vi "choose worker.vi"(9 "total":i32, 10 "Python version":string, 11 "user.xls path":path) -> ()   [LabVIEW 2020]
uses:
  status/emergency stop.vi
  status/experiment_No.vi
  status/status of worker1.vi
  status/pause1.vi
  status/status of worker2.vi
  status/pause2.vi
  status/status of worker3.vi
  status/pause3.vi
  status/pause4.vi
  status/status of worker4.vi
  status/stop software.vi
panel:
  in  "?":bool
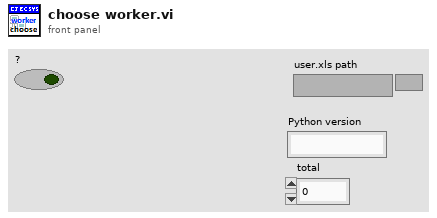
[diagram p1: front panel]
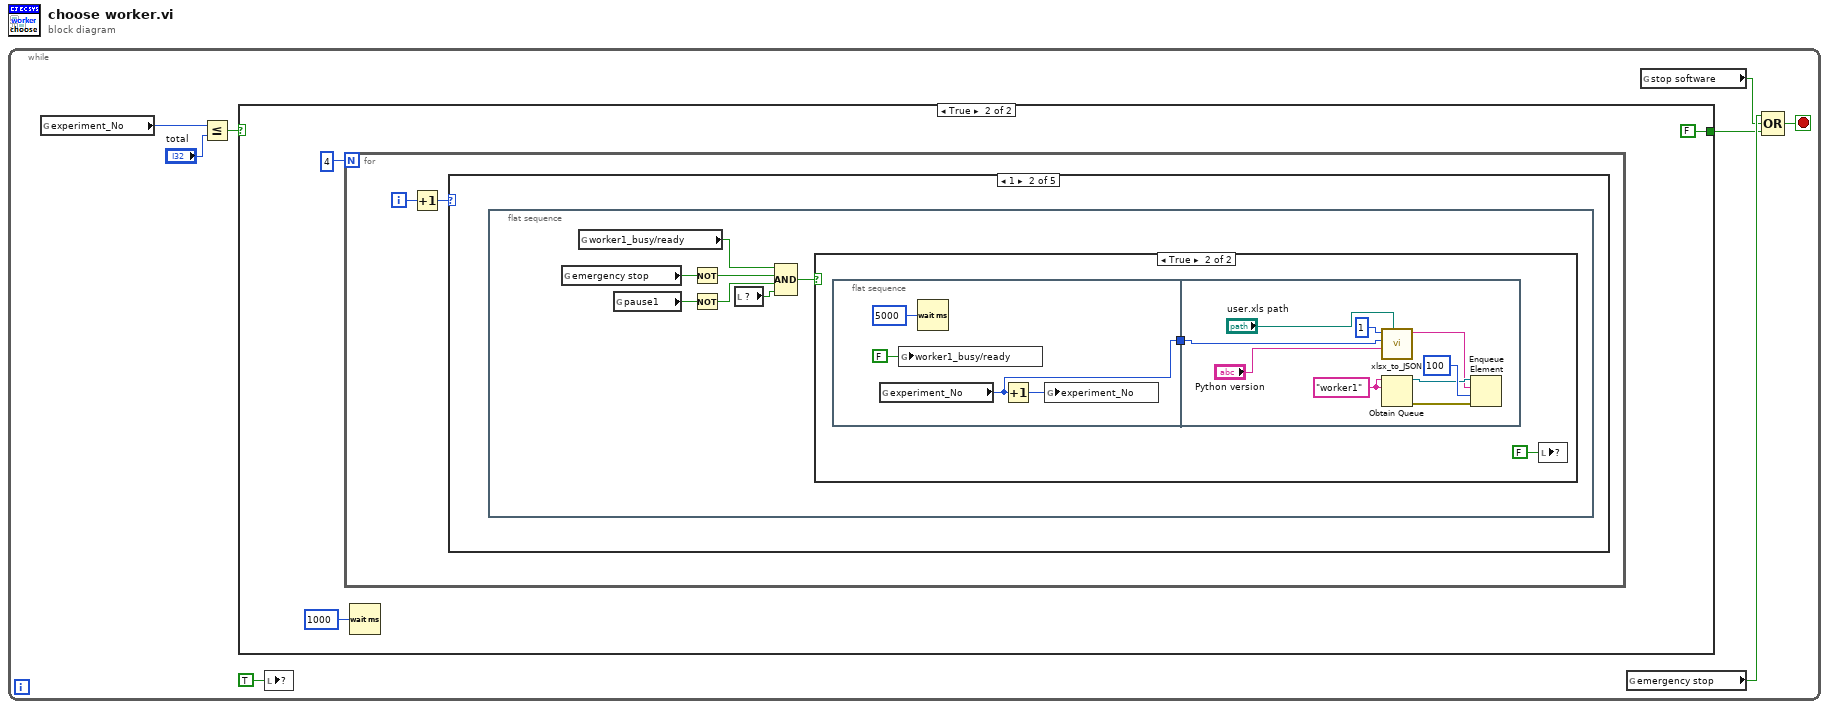
[diagram p0: block diagram]
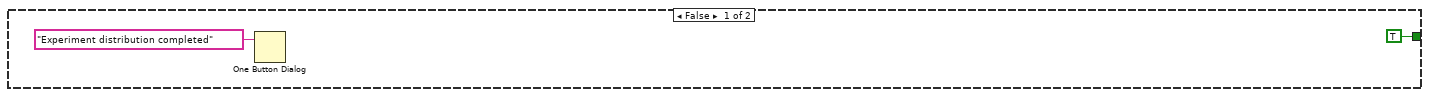
[diagram p2: hidden frame]
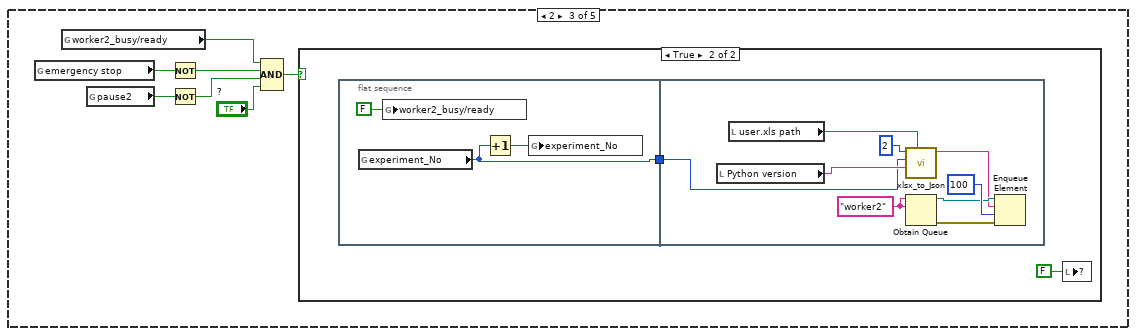
[diagram p5: hidden frame]
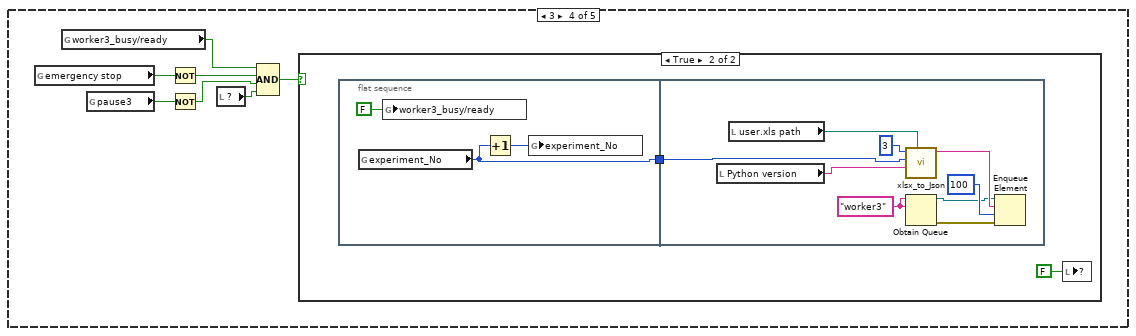
[diagram p7: hidden frame]
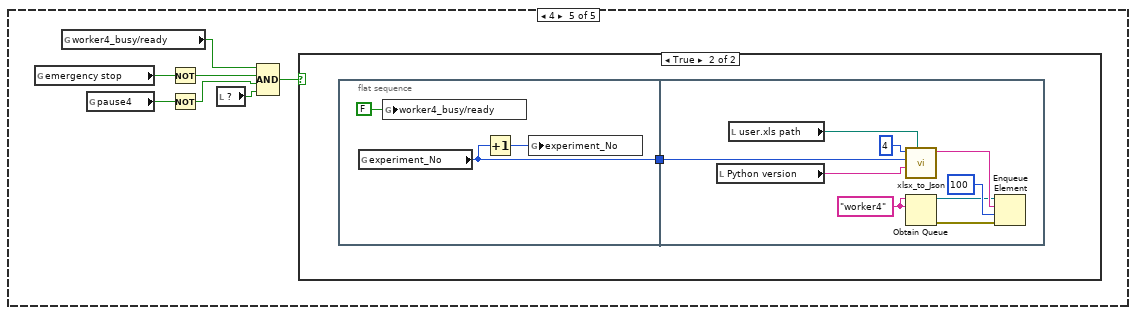
[diagram p9: hidden frame]
diagram:
  n1 = while {
    stop <- w1 stop-if-true
    n2 = global read "experiment_No.vi" "experiment_No"() -> (w6:i32)
    n3 = Less Or Equal?(x=w6, y="total") -> (x <= y?=w8:bool)
    n4 = case shown="True" w8 {
      tunnel: [TRUE FALSE] -> w2
      frame False {
        n5 = One Button Dialog(message="Experiment distribution completed") -> ()  [unwired: 1 in, 1 out]
      }
      frame True {
        n6 = for {
          N: 4 -> [_]
          i -> [w15]
          n7 = Increment(x=w15) -> (x+1=w14:i32)
          n8 = case shown="1" w14 {
            frame 0, Default {
            }
            frame 1 {
              n9 = flat-sequence {
                frame #0 {
                  n10 = global read "emergency stop.vi" "emergency stop"() -> (w22:bool)
                  n11 = global read "status of worker1.vi" "worker1_busy/ready"() -> (w20:bool)
                  n12 = global read "pause1.vi" "pause1"() -> (w21:bool)
                  n13 = Not(x=w22) -> (.not. x?=w19:bool)
                  n14 = Not(x=w21) -> (.not. x?=w18:bool)
                  n15 = local read "?"() -> (w16:bool)
                  n16 = Compound Arithmetic op=AND(w20, w19, w18, w16) -> (w17:bool)
                  n17 = case shown="True" w17 {
                    frame False {
                    }
                    frame True {
                      n18 = flat-sequence {
                        tunnel: [w26] -> w23
                        tunnel: w23 -> [w31]
                        frame #0 {
                          n19 = global read "experiment_No.vi" "experiment_No"() -> (w26:i32)
                          n20 = global write "status of worker1.vi" "worker1_busy/ready"(FALSE ("worker1_busy/ready")) -> ()
                          n21 = Wait (ms)(milliseconds to wait=u32 5000) -> ()  [unwired: 1 out]
                          n22 = Increment(x=w26) -> (x+1=w27:i32)
                          n23 = global write "experiment_No.vi" "experiment_No"(w27) -> ()
                        }
                        frame #1 {
                          w36 = "worker1" ("name (unnamed)")
                          n24 = call "xlsx_to_JSON.vi"("user.xls path"="user.xls path", "Python version"="Python version", "experiment_no"=w31, "worker_ID"=1) -> ("return value"=w29:string)  [unwired: 6 in, 1 out]
                          n25 = Obtain Queue(name (unnamed)=w36, element data type=w36) -> (queue out=w35:refnum<queue>, error out=w34:errorcluster)  [unwired: 3 in, 1 out]
                          n26 = Enqueue Element(queue=w35, element=w29, timeout in ms (-1)=100, error in (no error)=w34) -> ()  [unwired: 3 out]
                        }
                      }
                      n27 = local write "?"(FALSE ("?")) -> ()
                    }
                  }
                }
              }
            }
            frame 2 {
              n28 = global read "emergency stop.vi" "emergency stop"() -> (w44:bool)
              n29 = global read "status of worker2.vi" "worker2_busy/ready"() -> (w42:bool)
              n30 = global read "pause2.vi" "pause2"() -> (w40:bool)
              n31 = Not(x=w44) -> (.not. x?=w41:bool)
              n32 = Not(x=w40) -> (.not. x?=w39:bool)
              n33 = Compound Arithmetic op=AND(w42, w41, w39, "?") -> (w43:bool)
              n34 = case shown="True" w43 {
                frame False {
                }
                frame True {
                  n35 = flat-sequence {
                    tunnel: [w47] -> w46
                    tunnel: w46 -> [w53]
                    frame #0 {
                      n36 = global read "experiment_No.vi" "experiment_No"() -> (w47:i32)
                      n37 = global write "status of worker2.vi" "worker2_busy/ready"(FALSE ("worker1_busy/ready")) -> ()
                      n38 = Increment(x=w47) -> (x+1=w48:i32)
                      n39 = global write "experiment_No.vi" "experiment_No"(w48) -> ()
                    }
                    frame #1 {
                      w57 = "worker2" ("name (unnamed)")
                      n40 = local read "Python version"() -> (w54:string)
                      n41 = local read "user.xls path"() -> (w50:path)
                      n42 = call "xlsx_to_Json.vi"("user.xls path"=w50, "Python version"=w54, "experiment_no"=w53, "worker_ID"=2) -> ("return value"=w51:string)  [unwired: 6 in, 1 out]
                      n43 = Obtain Queue(name (unnamed)=w57, element data type=w57) -> (queue out=w56:refnum<queue>, error out=w55:errorcluster)  [unwired: 3 in, 1 out]
                      n44 = Enqueue Element(queue=w56, element=w51, timeout in ms (-1)=100, error in (no error)=w55) -> ()  [unwired: 3 out]
                    }
                  }
                  n45 = local write "?"(FALSE ("?")) -> ()
                }
              }
            }
            frame 3 {
              n46 = global read "emergency stop.vi" "emergency stop"() -> (w65:bool)
              n47 = global read "status of worker3.vi" "worker3_busy/ready"() -> (w60:bool)
              n48 = global read "pause3.vi" "pause3"() -> (w59:bool)
              n49 = Not(x=w65) -> (.not. x?=w63:bool)
              n50 = Not(x=w59) -> (.not. x?=w62:bool)
              n51 = local read "?"() -> (w61:bool)
              n52 = Compound Arithmetic op=AND(w60, w63, w62, w61) -> (w64:bool)
              n53 = case shown="True" w64 {
                frame False {
                }
                frame True {
                  n54 = flat-sequence {
                    tunnel: [w68] -> w67
                    tunnel: w67 -> [w76]
                    frame #0 {
                      n55 = global read "experiment_No.vi" "experiment_No"() -> (w68:i32)
                      n56 = global write "status of worker3.vi" "worker3_busy/ready"(FALSE ("worker1_busy/ready")) -> ()
                      n57 = Increment(x=w68) -> (x+1=w70:i32)
                      n58 = global write "experiment_No.vi" "experiment_No"(w70) -> ()
                    }
                    frame #1 {
                      w73 = "worker3" ("name (unnamed)")
                      n59 = local read "Python version"() -> (w75:string)
                      n60 = local read "user.xls path"() -> (w74:path)
                      n61 = call "xlsx_to_Json.vi"("user.xls path"=w74, "Python version"=w75, "experiment_no"=w76, "worker_ID"=3) -> ("return value"=w78:string)  [unwired: 6 in, 1 out]
                      n62 = Obtain Queue(name (unnamed)=w73, element data type=w73) -> (queue out=w72:refnum<queue>, error out=w71:errorcluster)  [unwired: 3 in, 1 out]
                      n63 = Enqueue Element(queue=w72, element=w78, timeout in ms (-1)=100, error in (no error)=w71) -> ()  [unwired: 3 out]
                    }
                  }
                  n64 = local write "?"(FALSE ("?")) -> ()
                }
              }
            }
            frame 4 {
              n65 = global read "emergency stop.vi" "emergency stop"() -> (w86:bool)
              n66 = global read "status of worker4.vi" "worker4_busy/ready"() -> (w80:bool)
              n67 = global read "pause4.vi" "pause4"() -> (w81:bool)
              n68 = Not(x=w86) -> (.not. x?=w84:bool)
              n69 = Not(x=w81) -> (.not. x?=w83:bool)
              n70 = local read "?"() -> (w82:bool)
              n71 = Compound Arithmetic op=AND(w80, w84, w83, w82) -> (w85:bool)
              n72 = case shown="True" w85 {
                frame False {
                }
                frame True {
                  n73 = flat-sequence {
                    tunnel: [w89] -> w87
                    tunnel: w87 -> [w96]
                    frame #0 {
                      n74 = global read "experiment_No.vi" "experiment_No"() -> (w89:i32)
                      n75 = global write "status of worker4.vi" "worker4_busy/ready"(FALSE ("worker1_busy/ready")) -> ()
                      n76 = Increment(x=w89) -> (x+1=w90:i32)
                      n77 = global write "experiment_No.vi" "experiment_No"(w90) -> ()
                    }
                    frame #1 {
                      w93 = "worker4" ("name (unnamed)")
                      n78 = local read "Python version"() -> (w95:string)
                      n79 = local read "user.xls path"() -> (w94:path)
                      n80 = call "xlsx_to_Json.vi"("user.xls path"=w94, "Python version"=w95, "experiment_no"=w96, "worker_ID"=4) -> ("return value"=w98:string)  [unwired: 6 in, 1 out]
                      n81 = Obtain Queue(name (unnamed)=w93, element data type=w93) -> (queue out=w92:refnum<queue>, error out=w91:errorcluster)  [unwired: 3 in, 1 out]
                      n82 = Enqueue Element(queue=w92, element=w98, timeout in ms (-1)=100, error in (no error)=w91) -> ()  [unwired: 3 out]
                    }
                  }
                }
              }
            }
          }
        }
        n83 = Wait (ms)(milliseconds to wait=u32 1000) -> ()  [unwired: 1 out]
      }
    }
    n84 = local write "?"(TRUE ("?")) -> ()
    n85 = global read "emergency stop.vi" "emergency stop"() -> (w4:bool)
    n86 = global read "stop software.vi" "stop software"() -> (w3:bool)
    n87 = Compound Arithmetic op=OR(w4, w3, w2) -> (w1:bool)
  }
